vi "read_lidar.vi"() -> ()   [LabVIEW 2016]
uses:
  Type Definitions/Controls/Measurement Parameters.ctl
  Type Definitions/Controls/Measurement Type.ctl
  <vilib>/Analysis/baseanly.llb/Mean (DBL).vi
  <vilib>/imath/engines/lvmath2/RunTimeEngine/BuiltInFunctions/linramp/NIMS_linramp.vi
  <vilib>/imath/engines/lvmath2/RunTimeEngine/IndexRead/NIMS V($).vi
  <instcachedir>/0/NIMS V($)_C593F32C7F6B43C7B1793952E292524F.lvgen/NIMS V($)_C593F32C7F6B43C7B1793952E292524F_001.vi
  <vilib>/imathl/engines/lvmath/Functions/Error Handling/Create Error.vi
  <vilib>/imath/engines/lvmath2/RunTimeEngine/IndexRead/NIMS V(R2).vi
  <instcachedir>/0/NIMS V(R2)_C76619605A0E4E9F8B2FA9389712AC47.lvgen/NIMS V(R2)_C76619605A0E4E9F8B2FA9389712AC47_000.vi
  <vilib>/imath/engines/lvmath2/RunTimeEngine/BuiltInFunctions/mirrorv/NIMS_mirrorv(GColV).vi
  <instcachedir>/0/NIMS_mirrorv(GColV)_C28FB1AB93194ED2915BC859B7BD4827.lvgen/NIMS_mirrorv(GColV)_C28FB1AB93194ED2915BC859B7BD4827_000.vi
  <vilib>/imath/engines/lvmath2/RunTimeEngine/NodeEndStatement/NIMS_NodeEndStatement_Output.vi
  <instcachedir>/0/NIMS_NodeEndStatement_Output_53EC0D466D134D7ABD903AC30B43404B.lvgen/NIMS_NodeEndStatement_Output_53EC0D466D134D7ABD903AC30B43404B_005.vi
  <vilib>/imath/engines/lvmath2/RunTimeEngine/ErrorHandling/NIMS_Finalize Error.vi
  <vilib>/Analysis/NI_AALBase.lvlib
panel:
  out "Waveform Chart":dbl(graph)
  out "Distance":dbl format="%0.2f"
  out "element 2":dbl
  out "element":dbl
  out "size(s)":i32
  in  "Hokuyo VISA Resource Reference":refnum<visa-resource-name>="USB0::0x15D1::0x0000::NI-VISA-1002::1::RAW"
  in  "Stop Test":bool
  out "Measurement Data":i32[](array[numeric])
  out "XY Graph":cluster{dbl, dbl}[](graph)
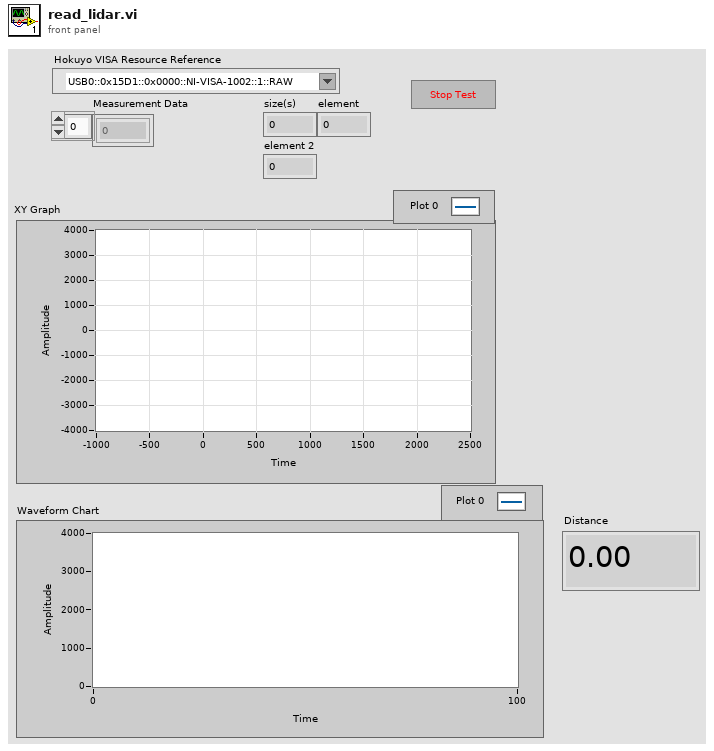
[diagram p1: front panel]
types:
  T1 = typedef "Measurement Parameters.ctl" = cluster{"Start Step":u32, "End Step":u32, "Cluster Count":u32, "Scan Interval":u32, "Number of Scans":u32, "Measurement Type":T2}
  T2 = typedef "Measurement Type.ctl" = enum16{"MS"}
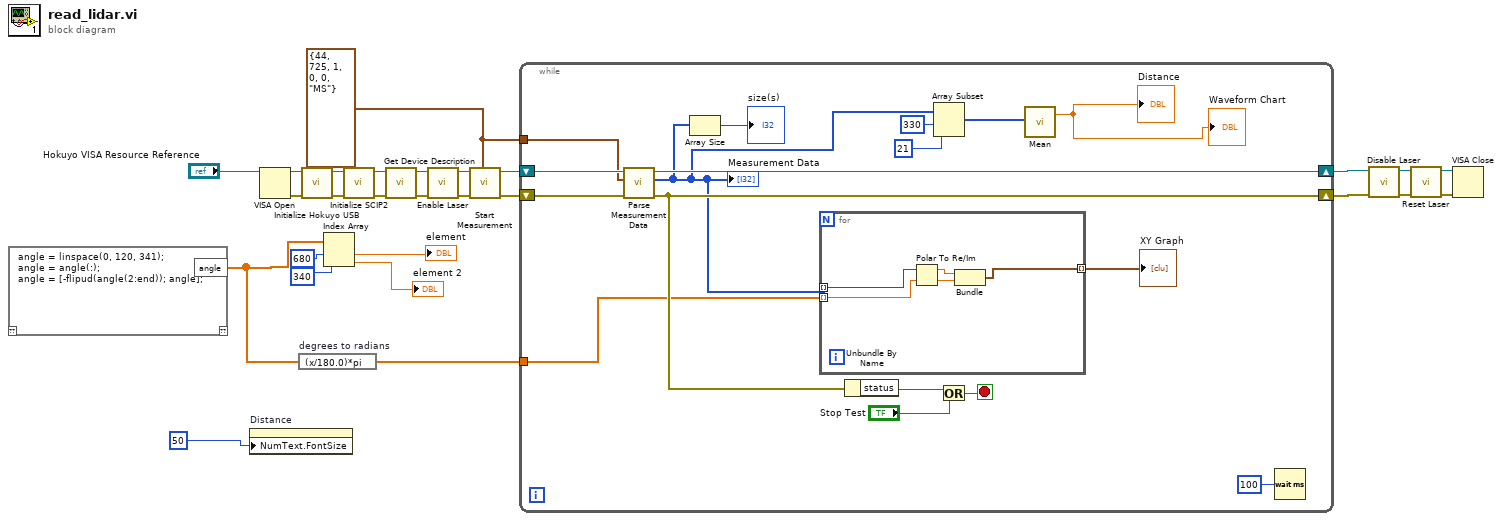
[diagram p0: block diagram]
diagram:
  w9 = T1 {"Start Step"=44, "End Step"=725, "Cluster Count"=1, "Scan Interval"=0, "Number of Scans"=0, "Measurement Type"=enum."MS"} ("Measurement Parameters")
  n1 = mathscript code="angle = linspace(0, 120, 341);\nangle = angle(:);\nangle = [-flipud(angle(2:end)); angle];"() -> ("angle"=w3:dbl[])  [unwired: 1 in, 1 out]
  n2 = property on="Distance" class="DigNum (strict)"("NumText.FontSize"=u32 50 ("Numeric Text.Size:Height")) -> ()  [unwired: 2 in, 2 out]
  n3 = VISA Open(VISA resource name="Hokuyo VISA Resource Reference") -> (VISA resource name=w17:refnum<visa-resource-name>, error out=w26:errorcluster)  [unwired: 4 in]
  n4 = expression code="(x/180.0)*pi" "degrees to radians"(w3) -> (w2:dbl[])
  n5 = call "Initialize Hokuyo USB.vi"("error in (no error)"=w26, "VISA Refnum in"=w17) -> ("error out"=w27:errorcluster, "VISA Refnum out"=w16:refnum<visa-resource-name>)  [unwired: 8 in]
  n6 = Index Array(array=w3, index #1=680 ("index"), index #2=340 ("index")) -> (element #1=→"element":dbl, element #2=→"element 2":dbl)
  n7 = call "Initialize SCIP2.vi"("error in (no error)"=w27, "VISA Refnum in"=w16) -> ("error out"=w24:errorcluster, "VISA Refnum out"=w15:refnum<visa-resource-name>)  [unwired: 8 in]
  n8 = call "Get Device Description.vi"("error in (no error)"=w24, "VISA Refnum in"=w15) -> ("error out"=w25:errorcluster, "VISA Refnum out"=w14:refnum<visa-resource-name>)  [unwired: 7 in, 1 out]
  n9 = call "Enable Laser.vi"("error in (no error)"=w25, "VISA Refnum in"=w14) -> ("error out"=w21:errorcluster, "VISA Refnum out"=w13:refnum<visa-resource-name>)  [unwired: 8 in]
  n10 = call "Start Measurement.vi"("error in (no error)"=w21, "Measurement Parameters"=w9, "VISA Refnum in"=w13) -> ("error out"=w20:errorcluster, "VISA Refnum out"=w12:refnum<visa-resource-name>)  [unwired: 7 in]
  n11 = while {
    tunnel: w9 -> [w41]
    shift-right: [w42] -> w11
    shift-left: w12 -> [w43]
    shift-right: [w39] -> w19
    shift-left: w20 -> [w44]
    tunnel: w2 -> [w33]
    stop <- w37 stop-if-true
    n12 = call "Parse Measurement Data.vi"("error in (no error)"=w44, "Measurement Parameters"=w41, "VISA Refnum in"=w43) -> ("error out"=w39:errorcluster, "Measurement Data"=w32:i32[], "VISA Refnum out"=w42:refnum<visa-resource-name>)  [unwired: 6 in]
    "Measurement Data" <- w32
    n13 = Array Size(array=w32) -> (size(s)=→"size(s)":i32)
    n14 = for {
      tunnel: w32 -> [w48] mode=indexing
      tunnel: [w49] -> w35 mode=indexing
      tunnel: w33 -> [w45] mode=indexing
      n15 = Polar To Re/Im(2:w45, 3:w48) -> (0:w46:dbl, 1:w47:dbl)
      n16 = Bundle(w47, w46) -> (w49:cluster{dbl, dbl})  [unwired: 1 in]
    }
    "XY Graph" <- w35
    n17 = Unbundle By Name(w39) -> ("status"=w38:bool)
    n18 = Array Subset(array=w32, index=330, length=21) -> (w29:i32[])
    n19 = Or(x=w38, y="Stop Test") -> (x .or. y?=w37:bool)
    n20 = call-poly <vilib>:"Mean.vi"("X"=w29) -> ("mean"=→"Distance" →"Waveform Chart":dbl)  [unwired: 1 out]
    n21 = Wait (ms)(milliseconds to wait=u32 100) -> ()  [unwired: 1 out]
  }
  n22 = call "Disable Laser.vi"("error in (no error)"=w19, "VISA Refnum in"=w11) -> ("error out"=w23:errorcluster, "VISA Refnum out"=w10:refnum<visa-resource-name>)  [unwired: 8 in]
  n23 = call "Reset Laser.vi"("error in (no error)"=w23, "VISA Refnum in"=w10) -> ("error out"=w22:errorcluster, "VISA Refnum out"=w8:refnum<visa-resource-name>)  [unwired: 8 in]
  n24 = VISA Close(VISA resource name=w8, error in (no error)=w22) -> ()  [unwired: 1 out]
